vi "initialize tree.vi"(7 "Filter in":refnum<class "Filter.lvclass">, 8 "error in (no error)":errorcluster, 10 "TreeControl in":refnum<vi>, 11 "Node Ptr":T1 format="%.0x") -> (0 "error out":errorcluster, 3 "Item Ref out":T1 format="%.0x")   [LabVIEW 2016, in "FPGA Resource Manager System Defintion.lvlib"]
uses:
  FPGA Resource Manager System Defintion.lvlib
  <vilib>/NI Veristand/Custom Device API/Custom Device Item Ref.ctl
  Filters/Filter Parent/Filter.lvclass
  reservation type.ctl
  viz_show.ctl
  <vilib>/NI Veristand/Custom Device API/Get Item Property (Dependent Node Pointer).vi
  <vilib>/NI Veristand/Custom Device API/Custom Device API.lvlib
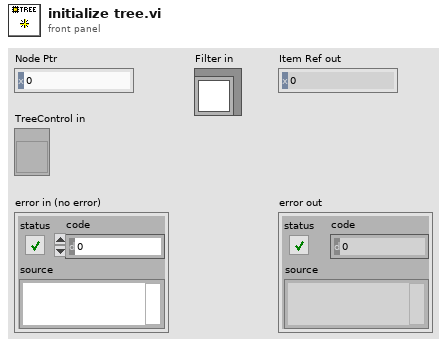
[diagram p1: front panel]
types:
  T1 = typedef "Custom Device API.lvlib/Custom Device Item Ref.ctl" = u64
  T2 = typedef "FPGA Resource Manager System Defintion.lvlib/viz_show.ctl" = enum16{"All", "Mapped", "Unmapped"}
  T3 = cluster{"Left Cell String":string, "Child Text":string[], "Child Tag":string, "Item Indent":i32, "Child Only?":bool, "Glyph Index":i32}[]
  T4 = typedef "FPGA Resource Manager System Defintion.lvlib/reservation type.ctl" = enum16{"none", "available", "reserved by this", "reserved by other", "incompatible", "parent"}
  T5 = typedef "FPGA Resource Manager System Defintion.lvlib/resource info.ctl" = cluster{"FPGA CD Ref":T1, "resource name":string, "input type":string, "datatype":string, "reserver":T1, "notes":string}
  T6 = cluster{"Left Cell String":string, "Child Text":string[], "Child Tag":string, "Item Indent":i32, "Child Only?":bool, "Glyph Index":i32}
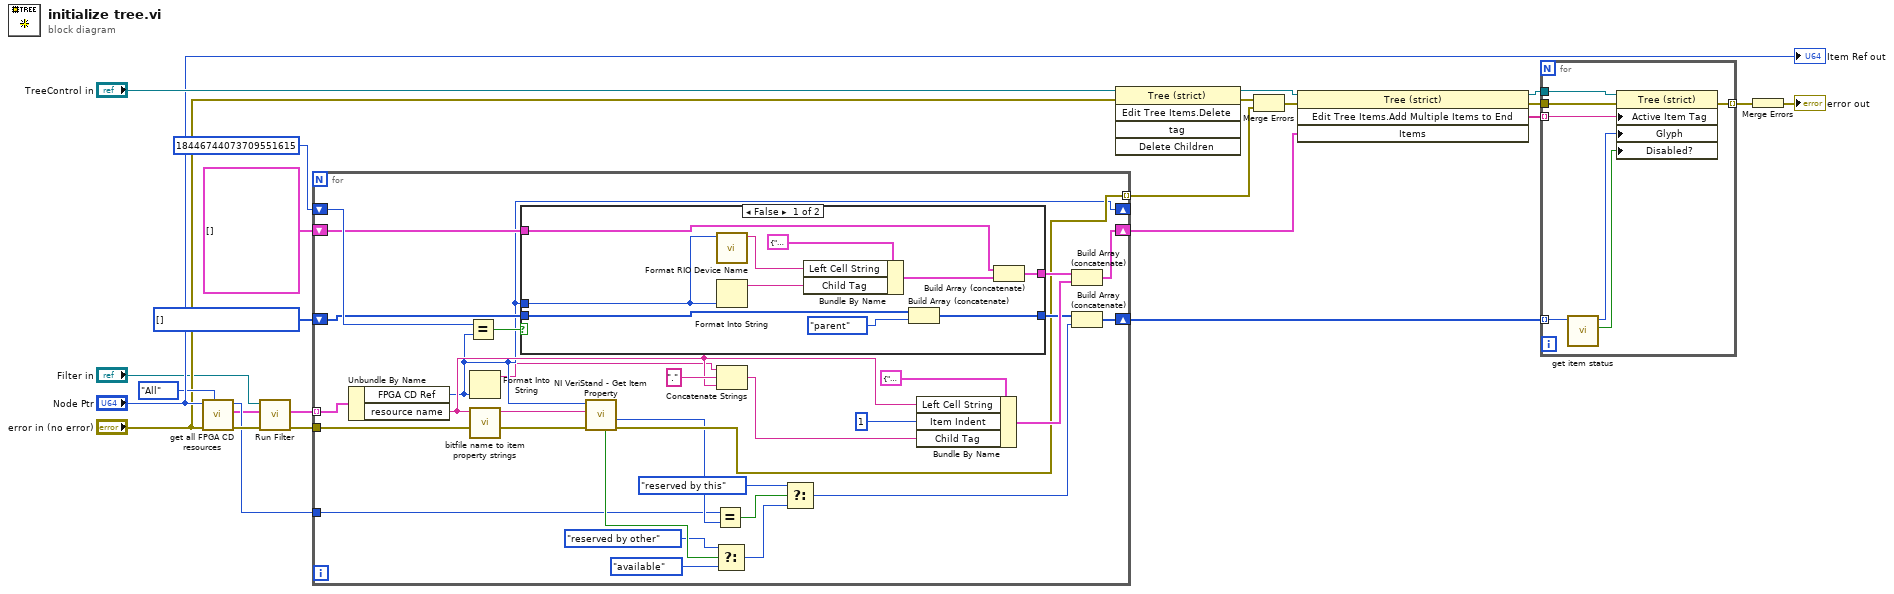
[diagram p0: block diagram]
diagram:
  w20 = T4[] [] items=["none", "available", "reserved by this", "reserved by other", "incompatible", "parent"]
  n1 = call "get all FPGA CD resources.vi"("Show"=viz_show."All", "error in (no error)"="error in (no error)", "Item Ref in"="Node Ptr") -> ("error out"=w12:errorcluster, "resource entries"=w3:T5[], "Item Ref out"=w5:T1)  [unwired: 6 in]
  n2 = call-dynamic "Run Filter.vi"("error in (no error)"=w12, "resource entries in"=w3, "Filter in"="Filter in") -> ("error out"=w4:errorcluster, "resource entries out"=w2:T5[])  [unwired: 7 in]
  n3 = for {
    tunnel: w2 -> [w53] mode=indexing
    shift-right: [w34] -> _
    shift-left: T1 18446744073709551615 ("FPGA CD Ref") -> [w51]
    shift-right: [w46] -> w18
    shift-left: T3 [] ("Item") -> [w49]
    shift-right: [w37] -> w16
    shift-left: w20 -> [w42]
    tunnel: w4 -> [w36]
    tunnel: [w35] -> w11 mode=indexing
    tunnel: w5 -> [w31]
    n4 = Unbundle By Name(w53) -> ("FPGA CD Ref"=w34:T1, "resource name"=w41:string)
    n5 = Equal?(x=w51, y=w34) -> (x = y?=w50:bool)
    n6 = Format Into String(w34) -> (resulting string=w33:string)  [unwired: 3 in, 1 out]
    n7 = call "bitfile name to item property strings.vi"("Name in bitfile"=w41) -> ("Reservation String"=w40:string)  [unwired: 9 in, 1 out]
    n8 = case shown="False" w50 {
      tunnel: w34 -> [w62 _]
      tunnel: w49 -> [w60 w65]
      tunnel: [w58 w65] -> w48
      tunnel: w42 -> [w56 w64]
      tunnel: [w55 w64] -> w38
      frame False {
        n9 = call "Format RIO Device Name.vi"("FPGA CD Ref"=w62) -> ("String"=w57:string)  [unwired: 9 in, 1 out]
        n10 = Format Into String(w62) -> (resulting string=w61:string)  [unwired: 3 in, 1 out]
        n11 = Bundle By Name(cluster=T6 {"Left Cell String"="", "Child Text"=[], "Child Tag"="", "Item Indent"=0, "Child Only?"=FALSE, "Glyph Index"=0} ("Item"), "Left Cell String"=w57, "Child Tag"=w61) -> (w59:T6)
        n12 = Build Array (concatenate)(w56, reservation_type."parent" ("element")) -> (w55:T4[])
        n13 = Build Array (concatenate)(w60, w59) -> (w58:T3)
      }
      frame True {
      }
    }
    n14 = call-poly <vilib>:"NI VeriStand - Get Item Property.vi"("error in (no error)"=w36, "Property Name"=w40, "Item Ref in"=w34) -> ("error out"=w35:errorcluster, "Dependent Node Ref"=w32:T1, "Found"=w39:bool)  [unwired: 5 in, 1 out]
    n15 = Equal?(x=w31, y=w32) -> (x = y?=w30:bool)
    n16 = Select(t=reservation_type."reserved by other" ("element"), s=w39, f=reservation_type."available" ("element")) -> (s? t:f=w26:T4)
    n17 = Concatenate Strings(w33, "." ("string"), w41) -> (w43:string)
    n18 = Select(t=reservation_type."reserved by this" ("element"), s=w30, f=w26) -> (s? t:f=w25:T4)
    n19 = Bundle By Name(cluster=T6 {"Left Cell String"="", "Child Text"=[], "Child Tag"="", "Item Indent"=0, "Child Only?"=FALSE, "Glyph Index"=0} ("Item"), "Left Cell String"=w41, "Item Indent"=1, "Child Tag"=w43) -> (w47:T6)
    n20 = Build Array (concatenate)(w48, w47) -> (w46:T3)
    n21 = Build Array (concatenate)(w38, w25) -> (w37:T4[])
  }
  n22 = invoke on="Invoke Node" class="Tree (strict)" method="Edit Tree Items.Delete"(reference="TreeControl in", error in="error in (no error)") -> (reference out=w19:refnum<vi>, error out=w10:errorcluster)  [unwired: 3 in, 3 out]
  n23 = Merge Errors(w10, w11) -> (w9:errorcluster)
  n24 = invoke on="Invoke Node" class="Tree (strict)" method="Edit Tree Items.Add Multiple Items to End"(reference=w19, error in=w9, "Items"=w18) -> (reference out=w15:refnum<vi>, error out=w8:errorcluster, "Edit Tree Items:Add Multiple Items to End"=w17:string[])  [unwired: 1 in, 1 out]
  n25 = for {
    tunnel: w17 -> [w72] mode=indexing
    tunnel: w16 -> [w71] mode=indexing
    tunnel: w15 -> [w68]
    tunnel: w8 -> [w67]
    tunnel: [w66] -> w7 mode=indexing
    n26 = call "get item status.vi"("element"=w71) -> ("Disabled?"=w69:bool, "symbol index"=w70:i32)  [unwired: 9 in]
    n27 = property class="Tree (strict)"(reference=w68, error in=w67, "Active Item Tag"=w72, "Glyph"=w70, "Disabled?"=w69) -> (error out=w66:errorcluster)  [unwired: 1 out]
  }
  n28 = Merge Errors(w7) -> (→"error out":errorcluster)
  "Item Ref out" <- "Node Ptr"
